vi "Configure Load.vi"(8 "error in (no error)":errorcluster, 10 "Load Type (0: Low Impedance)":enum16{"Low Impedance", "High Impedance"}(ring), 11 "VISA resource name":refnum<visa-resource-name>) -> (0 "error out":errorcluster, 3 "VISA resource name out":refnum<visa-resource-name>)   [LabVIEW 2017, in "Keithley 3390.lvlib"]
doc: "Configures the function generator to adjust output to the proper level for the given load."
uses:
  Keithley 3390.lvlib
panel:
  in  "Impedance (50 Ohms)":i32=50 min=1 max=10000
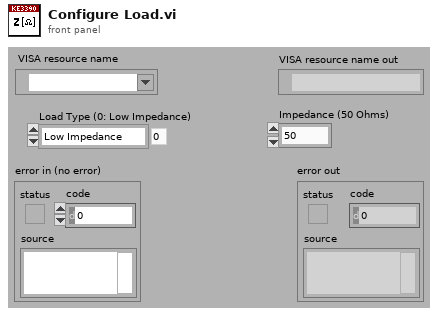
[diagram p1: front panel]
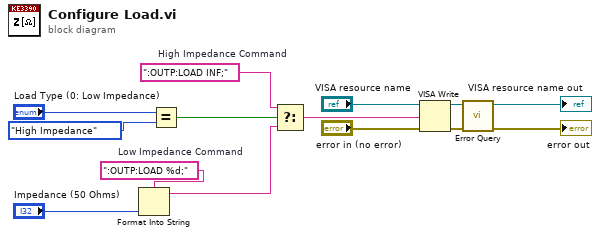
[diagram p0: block diagram]
diagram:
  w1 = ":OUTP:LOAD %d;"  # Low Impedance Command
  w4 = ":OUTP:LOAD INF;"  # High Impedance Command
  n1 = Format Into String(format string=w1, "Impedance (50 Ohms)") -> (resulting string=w3:string)  [unwired: 2 in, 1 out]
  n2 = Equal?(x="Load Type (0: Low Impedance)", y=enum16{"Low Impedance", "High Impedance"}."High Impedance") -> (x = y?=w5:bool)
  n3 = Select(t=w4, s=w5, f=w3) -> (s? t:f=w2:string)
  n4 = VISA Write(VISA resource name="VISA resource name", write buffer=w2, error in (no error)="error in (no error)") -> (VISA resource name out=w10:refnum<visa-resource-name>, error out=w9:errorcluster)  [unwired: 1 out]
  n5 = call "Error Query.vi"("error in (no error)"=w9, "VISA resource name"=w10) -> ("error out"=→"error out":errorcluster, "VISA resource name out"=→"VISA resource name out":refnum<visa-resource-name>)  [unwired: 6 in, 2 out]
